vi "Format Image URL.vi"(0 "file name":string, 7 "output dir":path, 11 "image dir":path) -> (4 "image URL string":string)   [LabVIEW 2019, in "MD Generator.lvlib"]
uses:
  MD Generator.lvlib
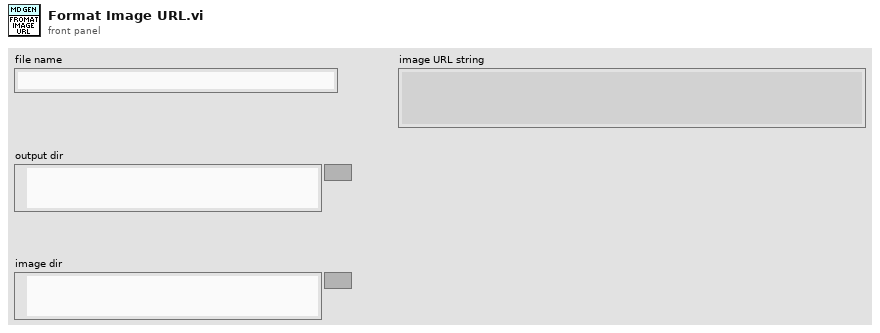
[diagram p1: front panel]
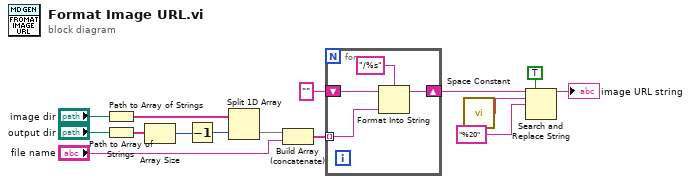
[diagram p0: block diagram]
diagram:
  n1 = Path to Array of Strings(0:"image dir") -> (2:w10:string[])  [unwired: 1 out]
  n2 = Path to Array of Strings(0:"output dir") -> (2:w11:string[])  [unwired: 1 out]
  n3 = Array Size(array=w11) -> (size(s)=w12:i32)
  n4 = Decrement(x=w12) -> (x-1=w1:i32)
  n5 = Split 1D Array(array=w10, index=w1) -> (second subarray=w9:string[])  [unwired: 1 out]
  n6 = Build Array (concatenate)(w9, "file name") -> (w7:string[])
  n7 = for {
    shift-right: [w18] -> w6
    shift-left: "" -> [w19]
    tunnel: w7 -> [w16] mode=indexing
    n8 = Format Into String(format string="/%s", initial string=w19, w16) -> (resulting string=w18:string)  [unwired: 1 in, 1 out]
  }
  n9 = call <vilib>:"Space Constant.vi"() -> ("String"=w5:string)
  n10 = Search and Replace String(replace all?=TRUE ("replace all? (F)"), input string=w6, search string=w5, replace string="%20" ("replace string (\"\")")) -> (result string=→"image URL string":string)  [unwired: 4 in, 3 out]
